vi "GetVisaRef.vi"(0 "reference in":refnum<class "VdRs232.lvclass">, 5 "error in (no error)":errorcluster) -> (14 "reference out":refnum<class "VdRs232.lvclass">, 15 "visaRef":refnum<visa-resource-name>="ASRL2::INSTR", 19 "error out":errorcluster)   [LabVIEW 2020, in "VdRs232.lvclass"]
uses:
  VdRs232.lvclass
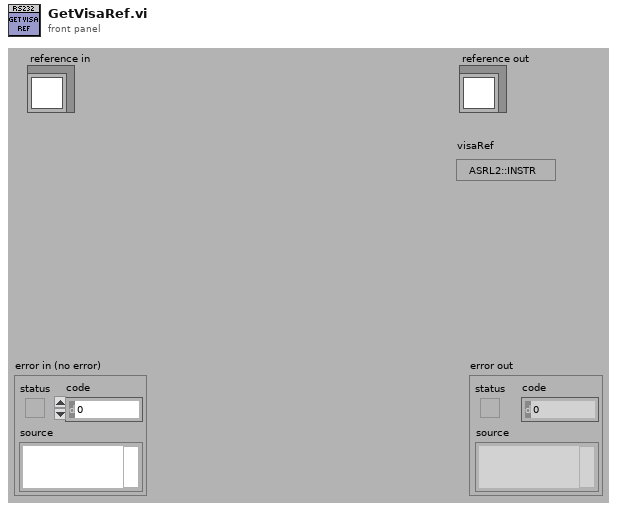
[diagram p1: front panel]
types:
  T1 = typedef "VdRs232.lvclass/ObjectAttributes.ctl" = cluster{"visaRef":refnum<visa-resource-name>, "portSetting":T2, "TimeoutTime(ms)":u32, "TerminationCharUsed":bool, "MatchPatternToIndicateCompleteResponse":string, "Creators":i32, "EndCharToSendForEveryMessage":string, "DefaultReadDataSize":u32, "SynchronousMode":bool, "Lock":T7}
  T2 = typedef "VdRs232.lvclass/ComParamsType.ctl" = cluster{"portNbr":T3, "baudRate":T4, "flowControl":T5, "parity":T6, "dataBits":u16, "stop bits (10: 1 bit)":u16}
  T3 = typedef "VdRs232.lvclass/VdRs232I_ComPortType.ctl" = enum16{"Com1", "Com2", "Com3", "Com4", "Com5", "Com6", "Com7", "Com8", "Com9", "Com10", "Com11", "Com12", "Com13", "Com14", "Com15", "Com16", "Com17", "Com18", "Com19", "Com20", "Com21", "Com22", "Com23", "Com24", "Com25", "Com26", "Com27", "Com28", "Com29", "Com30", "Com31", "Com32", "Com33", "Com34", "Com35", "Com36", "Com37", "Com38", "Com39", "Com40", "Com41", "Com42", "Com43", "Com44", "Com45", "Com46", "Com47", "Com48", "Com49", "Com50", "Com51", "Com52", "Com53", "Com54", "Com55", "Com56", "Com57", "Com58", "Com59", "Com60", "Com61", "Com62", "Com63", "Com64", "Com65", "Com66", "Com67", "Com68", "Com69", "Com70", "Com71", "Com72", "Com73", "Com74", "Com75", "Com76", "Com77", "Com78", "Com79", "Com80", "Com81", "Com82", "Com83", "Com84", "Com85", "Com86", "Com87", "Com88", "Com89", "Com90", "Com91", "Com92", "Com93", "Com94", "Com95", "Com96", "Com97", "Com98", "Com99", "Com100", "Com101", "Com102", "Com103", "Com104", "Com105", "Com106", "Com107", "Com108", "Com109", "Com110", "Com111", "Com112", "Com113", "Com114", "Com115", "Com116", "Com117", "Com118", "Com119", "Com120", "Com121", "Com122", "Com123", "Com124", "Com125", "Com126", "Com127", "Com128", "Com129", "Com130", "Com131", "Com132", "Com133", "Com134", "Com135", "Com136", "Com137", "Com138", "Com139", "Com140", "Com141", "Com142", "Com143", "Com144", "Com145", "Com146", "Com147", "Com148", "Com149", "Com150", "Com151", "Com152", "Com153", "Com154", "Com155", "Com156", "Com157", "Com158", "Com159", "Com160", "Com161", "Com162", "Com163", "Com164", "Com165", "Com166", "Com167", "Com168", "Com169", "Com170", "Com171", "Com172", "Com173", "Com174", "Com175", "Com176", "Com177", "Com178", "Com179", "Com180", "Com181", "Com182", "Com183", "Com184", "Com185", "Com186", "Com187", "Com188", "Com189", "Com190", "Com191", "Com192", "Com193", "Com194", "Com195", "Com196", "Com197", "Com198", "Com199", "Com200", "Com201", "Com202", "Com203", "Com204", "Com205", "Com206", "Com207", "Com208", "Com209", "Com210", "Com211", "Com212", "Com213", "Com214", "Com215", "Com216", "Com217", "Com218", "Com219", "Com220", "Com221", "Com222", "Com223", "Com224", "Com225", "Com226", "Com227", "Com228", "Com229", "Com230", "Com231", "Com232", "Com233", "Com234", "Com235", "Com236", "Com237", "Com238", "Com239", "Com240", "Com241", "Com242", "Com243", "Com244", "Com245", "Com246", "Com247", "Com248", "Com249", "Com250", "Com251", "Com252", "Com253", "Com254", "Com255"}
  T4 = typedef "VdRs232.lvclass/VdBaudRateType.ctl" = enum16{"1200", "2400", "9600", "14400", "19200", "28800", "38400", "57600", "115200", "230400", "460800", "691200", "921600"}
  T5 = typedef "VdRs232.lvclass/VdFlowControlType.ctl" = enum16{"None", "CTS/RTS", "XOn/XOff"}
  T6 = typedef "VdRs232.lvclass/VdParityType.ctl" = enum16{"None", "Odd", "Even"}
  T7 = typedef "Semaphore RefNum" = refnum<k1>
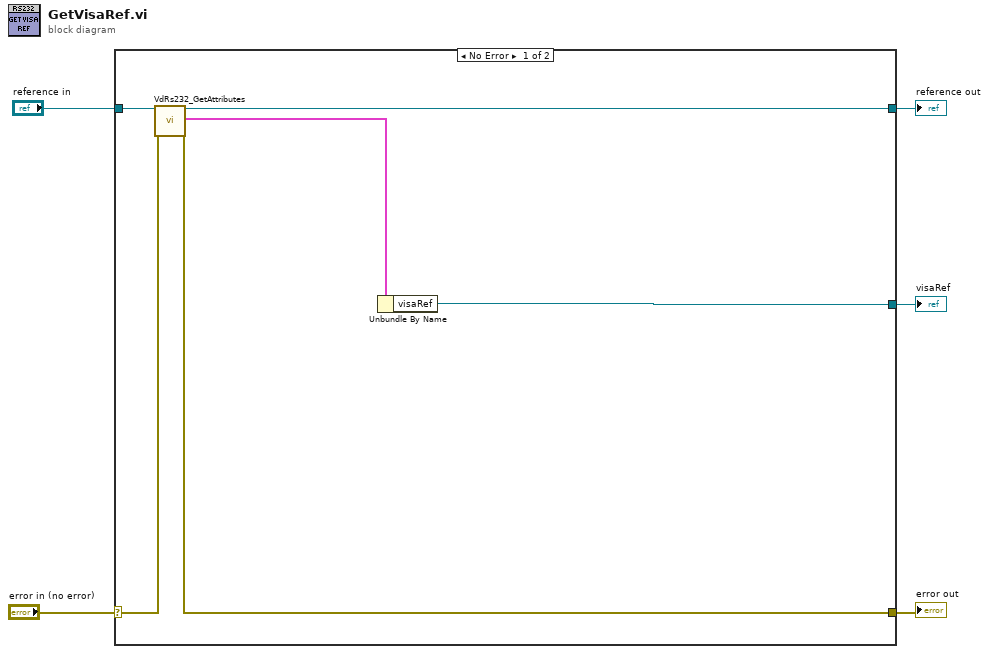
[diagram p0: block diagram]
diagram:
  n1 = case shown="No Error" "error in (no error)" {
    selector: "error in (no error)" -> [w11 w13]
    tunnel: [w10 w13] -> w4
    tunnel: [w8 w12] -> w2
    tunnel: "reference in" -> [w9 w12]
    tunnel: [w7 _] -> w1
    frame No Error {
      n2 = call "VdRs232_GetAttributes.vi"("reference in"=w9, "error in (no error)"=w11) -> ("reference out"=w8:refnum<class "VdRs232.lvclass">, "Data"=w6:T1, "error out"=w10:errorcluster)  [unwired: 14 in, 1 out]
      n3 = Unbundle By Name(w6) -> ("visaRef"=w7:refnum<visa-resource-name>)
    }
    frame Error {
    }
  }
  "error out" <- w4
  "reference out" <- w2
  "visaRef" <- w1
